vi "Write rtTimestamp.vi"(8 "error in (no error)":errorcluster, 10 "rtTimestamp":dbl, 11 "ComponentData in":refnum<class "ComponentData.lvclass">) -> (0 "error out":errorcluster, 3 "ComponentData out":refnum<class "ComponentData.lvclass">)   [LabVIEW 2013, in "ComponentData.lvlib" / "ComponentData.lvclass"]
uses:
  <userlib>/Common/Component/Application/RT/ComponentData/ComponentData/ComponentData.lvclass
  <userlib>/Common/Component/Application/RT/ComponentData/ComponentData/ComponentData.lvclass/ComponentData.ctl
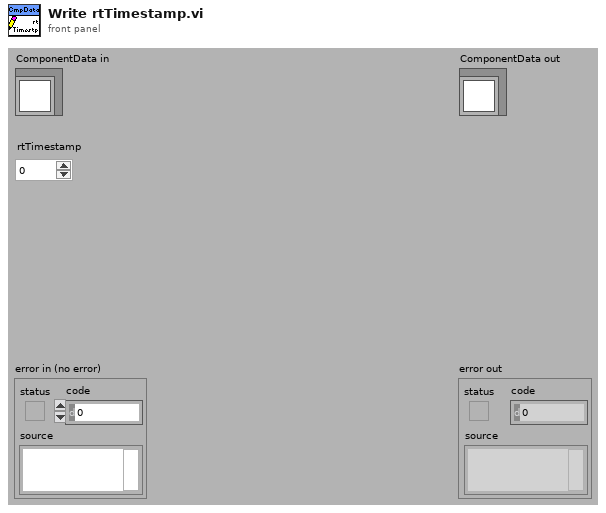
[diagram p1: front panel]
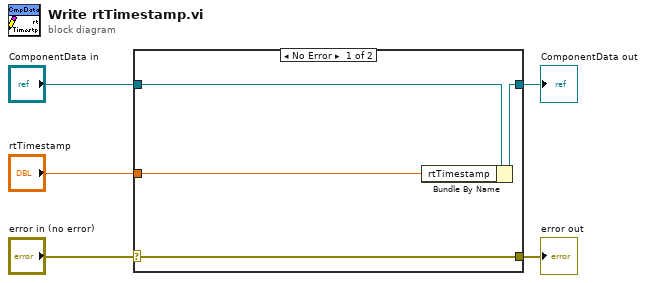
[diagram p0: block diagram]
diagram:
  n1 = case shown="No Error" "error in (no error)" {
    selector: "error in (no error)" -> [w9 w10]
    tunnel: [w9 w10] -> w4
    tunnel: [w7 w11] -> w2
    tunnel: "ComponentData in" -> [w8 w11]
    tunnel: "rtTimestamp" -> [w6 _]
    frame No Error {
      n2 = Bundle By Name(cluster=w8, "rtTimestamp"=w6) -> (w7:refnum<class "ComponentData.lvclass">)
    }
    frame Error {
    }
  }
  "error out" <- w4
  "ComponentData out" <- w2
